vi "oven_state_global.vi"() -> ()   [LabVIEW 2012]
panel:
  out "Oven State":bool
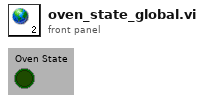
[diagram p1: front panel]
diagram:
